vi "Dash_HopperT_w_Rio.vi"() -> ()   [LabVIEW 2017, in "Hopper System.lvlib"]
uses:
  Hopper System.lvlib
  Cluster_CMD to SM Data.ctl
  ENUM_Firing_State.ctl
  Globals/Global_CMD to SM Data.vi
  Global_SM_Data Out.vi
  Global_HW Status.vi
  _SHARE ALL/Global Share All/Global_STOP.vi
panel:
  in  "Hopper_CMD":T1={"Enable Loading"=FALSE, "Disable Loading"=FALSE, "Fireing State"=enum."No Fireing", "Time Limit Loading"=5.0, "Time Limit Rapid"=2.0, "Rapid Fire Shot Limit"=3, "Shotgun Fire Shot Limit"=1}
  out "Hopper_SM_PercentVBus":dbl
  out "Hopper Line BallPresent":bool
  out "Hopper Line BallShot":bool
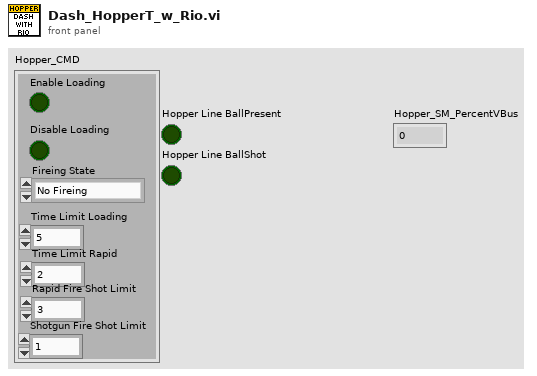
[diagram p1: front panel]
types:
  T1 = typedef "Hopper System.lvlib/Cluster_CMD to SM Data.ctl" = cluster{"Enable Loading":bool, "Disable Loading":bool, "Fireing State":T2, "Time Limit Loading":dbl, "Time Limit Rapid":dbl, "Rapid Fire Shot Limit":i32, "Shotgun Fire Shot Limit":i32}
  T2 = typedef "Hopper System.lvlib/ENUM_Firing_State.ctl" = enum16{"No Fireing", "Rapid Fire", "Shotgun Fireing"}
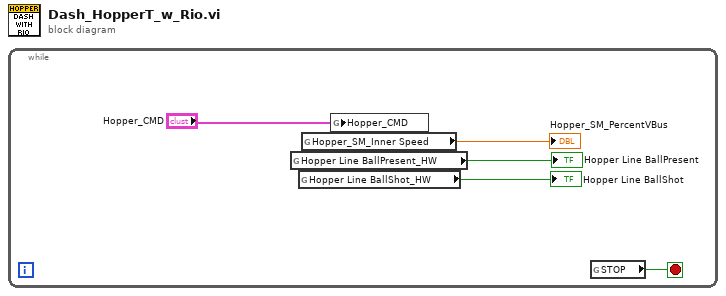
[diagram p0: block diagram]
diagram:
  n1 = while {
    stop <- w1 stop-if-true
    n2 = global read "Global_HW Status.vi" "Hopper Line BallPresent_HW"() -> (→"Hopper Line BallPresent":bool)
    n3 = global read "Global_HW Status.vi" "Hopper Line BallShot_HW"() -> (→"Hopper Line BallShot":bool)
    n4 = global read "Global_SM_Data Out.vi" "Hopper_SM_Inner Speed"() -> (→"Hopper_SM_PercentVBus":dbl)
    n5 = global write "Global_CMD to SM Data.vi" "Hopper_CMD"("Hopper_CMD") -> ()
    n6 = global read "Global_STOP.vi" "STOP"() -> (w1:bool)
  }
